vi "Reset Reference Oscillator.vi"(8 "error in (no error)":errorcluster, 11 "VISA resource name":refnum<visa-resource-name>) -> (0 "error out":errorcluster, 3 "VISA resource name out":refnum<visa-resource-name>)   [LabVIEW 2012, in "Agilent PSG MXG Series.lvlib"]
doc: "Resets the bandwidth of the reference oscillator to the factory-defined default state. The default value for the internal reference bandwidth is 125 Hz, and the default value for the external reference bandwidth is 25 Hz.\n\n<B>Notes:</B>\n(1) This VI is valid only in E8247C, E8257C, E8267C, E8257D, E8267D.\n\n(2) For E8247C, E8257C, E8267C, this VI is valid only when the instrument installs <B>Option UNR</B> (Enhanced phase noise performance).\n\n(3) For E8257D, E8267D, this VI is valid only when the instrument installs <B>Option UNR</B> or <B>Option UNX</B> (Ultra-low phase noise performance)."
uses:
  <instrlib>/Agilent PSG MXG Series/Agilent PSG MXG Series.lvlib
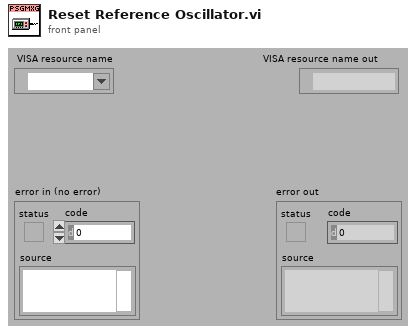
[diagram p1: front panel]
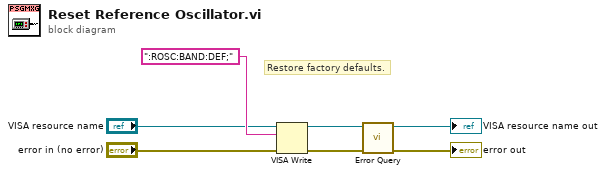
[diagram p0: block diagram]
diagram:
  # "Restore factory defaults."
  n1 = VISA Write(VISA resource name="VISA resource name", write buffer=":ROSC:BAND:DEF;", error in (no error)="error in (no error)") -> (VISA resource name out=w7:refnum<visa-resource-name>, error out=w6:errorcluster)  [unwired: 1 out]
  n2 = call <instrlib>:"Error Query.vi"("error in (no error)"=w6, "VISA resource name"=w7) -> ("error out"=→"error out":errorcluster, "VISA resource name out"=→"VISA resource name out":refnum<visa-resource-name>)  [unwired: 8 out]
